vi "HeaderAction.vi"(0 "DefaultDevIn":refnum<class "PhotoLum.lvclass"> caption="DNL_LabVIEW Object in", 11 "error in (no error)":errorcluster caption="entrée d'erreur (pas d'erreur)") -> (4 "DefaultDevOut":refnum<class "PhotoLum.lvclass"> caption="DNL_LabVIEW Object out", 6 "DataNames":string[](array[string]), 8 "Instr Name":string, 10 "HeaderString":string, 14 "DisplayNames":string[](array[string]), 15 "error out":errorcluster caption="sortie d'erreur")   [LabVIEW 2019, in "PhotoLum.lvclass"]
uses:
  PhotoLum.lvclass
  C:/Programmes Labview/LabScanV1A/DevicesClass/BaseDevice/BaseDevice.lvclass
  PhotoLum.lvclass/PhotoLum.ctl
  BaseDevice/BaseDevice.lvclass
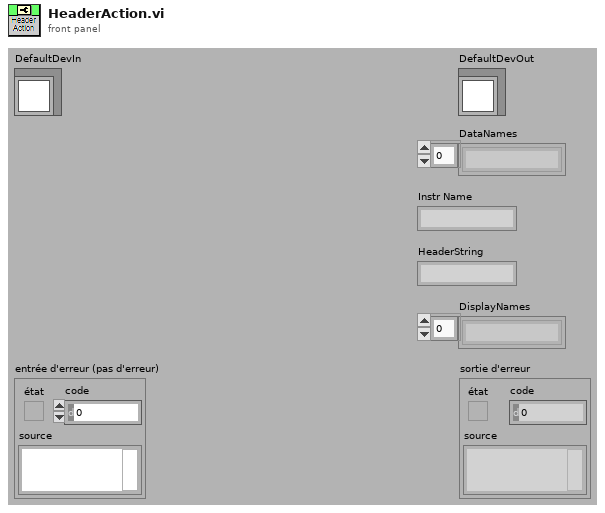
[diagram p1: front panel]
types:
  T1 = typedef "PhotoLum.lvclass/PhotoLum_Func.ctl" = enum16{"ScanInfoPanel (Na)", "MicroPLInfoPanel (NA)", "ExcimerInfoPan (NA)"}
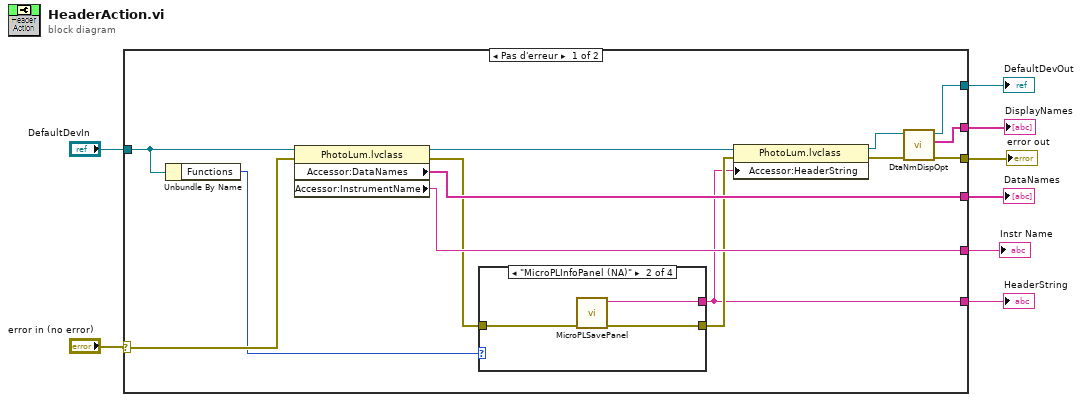
[diagram p0: block diagram]
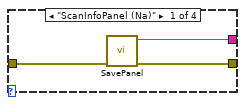
[diagram p2: hidden frame]
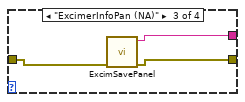
[diagram p3: hidden frame]
diagram:
  n1 = case shown="Pas d'erreur" "error in (no error)" {
    selector: "error in (no error)" -> [w22 w33]
    tunnel: [w21 _] -> w7
    tunnel: "DefaultDevIn" -> [w16 w34]
    tunnel: [w12 w33] -> w5
    tunnel: [w10 w34] -> w4
    tunnel: [w19 _] -> w3
    tunnel: [w14 _] -> w2
    tunnel: [w11 _] -> w1
    frame No Error {
      n2 = Unbundle By Name(w16) -> ("Functions"=w15:T1)
      n3 = property class="PhotoLum.lvclass"(reference=w16, error in=w22) -> (reference out=w20:refnum<class "PhotoLum.lvclass">, error out=w17:errorcluster, "Accessor:DataNames"=w21:string[], "Accessor:InstrumentName"=w19:string)
      n4 = case shown="\"MicroPLInfoPanel (NA)\"" w15 {
        tunnel: [w25 w28 w29 _] -> w14
        tunnel: w17 -> [w24 w27 w30 w32]
        tunnel: [w23 w26 w31 w32] -> w18
        frame "ScanInfoPanel (Na)" {
          n5 = call "SavePanel.vi"("error in"=w24) -> ("error out"=w23:errorcluster, "Chaîne"=w25:string)  [unwired: 9 in]
        }
        frame "MicroPLInfoPanel (NA)" {
          n6 = call "MicroPLSavePanel.vi"("error in"=w27) -> ("error out"=w26:errorcluster, "Chaîne"=w28:string)  [unwired: 9 in]
        }
        frame "ExcimerInfoPan (NA)" {
          n7 = call "ExcimSavePanel.vi"("error in"=w30) -> ("error out"=w31:errorcluster, "Chaîne"=w29:string)  [unwired: 9 in]
        }
        frame Default {
        }
      }
      n8 = property class="PhotoLum.lvclass"(reference=w20, error in=w18, "Accessor:HeaderString"=w14) -> (reference out=w9:refnum<class "PhotoLum.lvclass">, error out=w13:errorcluster)
      n9 = call "DtaNmDispOpt.vi"("error in (no error)"=w13, "BaseDevice en entrée"=w9) -> ("error out"=w12:errorcluster, "DisplayNames"=w11:string[], "BaseDevice en sortie"=w10:refnum<class "PhotoLum.lvclass">)  [unwired: 7 in]
    }
    frame Error {
    }
  }
  "error out" <- w5
  "DefaultDevOut" <- w4
  "DataNames" <- w7
  "HeaderString" <- w2
  "Instr Name" <- w3
  "DisplayNames" <- w1
